vi "opc_client.vi"(8 "error in (no error)":errorcluster, 10 "server endpoint URL":string) -> (0 "error out":errorcluster, 1 "OPC UA client refnum out":T1, 2 "etat":string, 3 "temperature":dbl, 4 "Courant":dbl, 5 "Pression":dbl, 6 "Debit":dbl, 7 "Tension":dbl)   [LabVIEW 2019]
uses:
  <vilib>/OPCUA/controls/OPC UA Client Refnum.ctl
  <vilib>/OPCUA/controls/Time Out.ctl
  <vilib>/OPCUA/client/Multiple Read Variant.vi
  <vilib>/OPCUA/NI OPC UA Client.lvlib
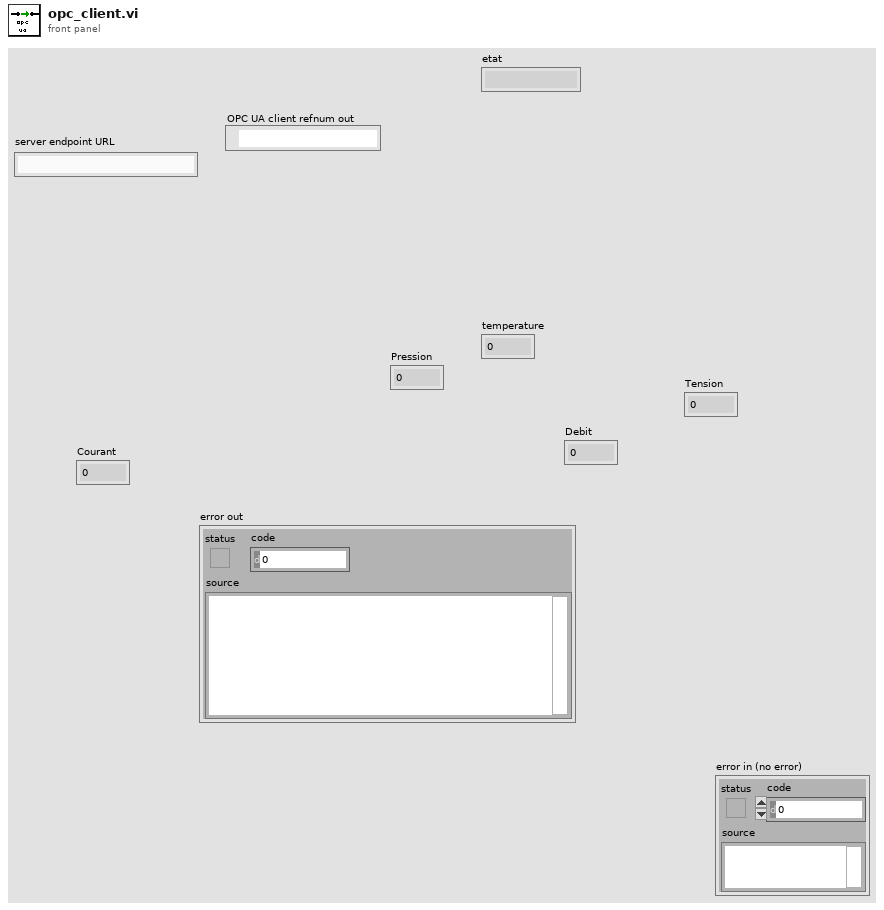
[diagram p1: front panel]
types:
  T1 = typedef "OPC UA Client Refnum.ctl" = refnum<k21>
  T2 = typedef "Time Out.ctl" = u32
  T3 = cluster{"message mode":enum16{"None", "Sign", "Sign and Encrypt"}, "security":enum16{"Basic256", "Basic128Rsa15"}}
  T4 = typedef "Read Variant Result.ctl" = cluster{"node ID":T5, "value ":variant, "timestamp":timestamp, "status":T6}
  T5 = typedef "NodeId.ctl" = string
  T6 = typedef "OPC UA StatusCode.ctl" = u32
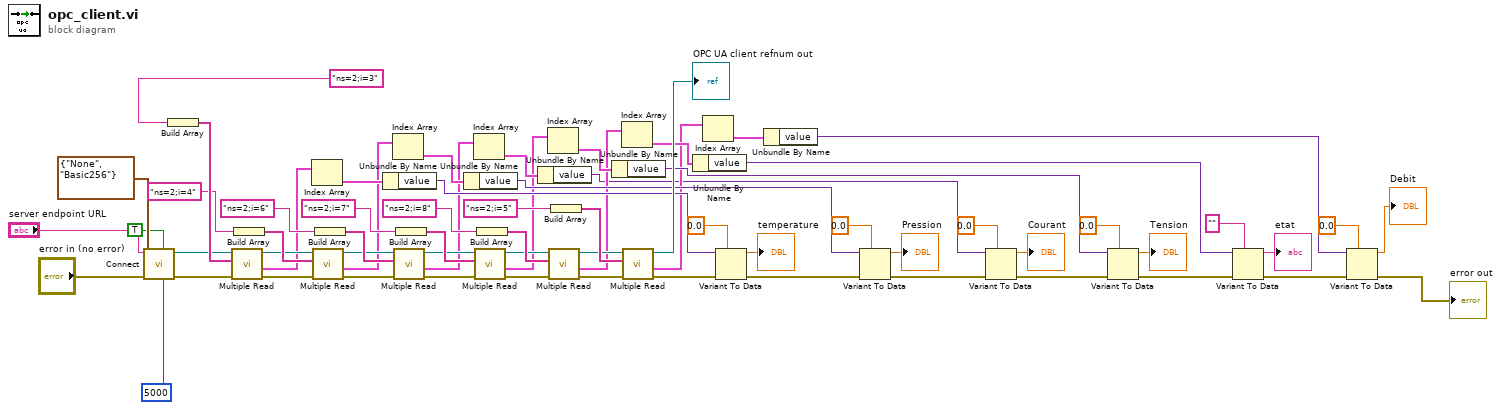
[diagram p0: block diagram]
diagram:
  n1 = call <vilib>:"Connect.vi"("timeout (5000 ms)"=T2 5000, "trust any server (F)"=TRUE, "error in (no error)"="error in (no error)", "security policy"=T3 {"message mode"=enum."None", "security"=enum."Basic256"}, "server endpoint URL"="server endpoint URL") -> ("error out"=w51:errorcluster, "OPC UA client refnum out"=w65:T1)  [unwired: 4 in, 1 out]
  n2 = Build Array("ns=2;i=3" ("ID")) -> (w66:string[])
  n3 = call-poly <vilib>:"Multiple Read.vi"("error in (no error)"=w51, "node IDs"=w66, "OPC UA client refnum in"=w65) -> ("error out"=w50:errorcluster, "results"=w40:T4[], "OPC UA client refnum out"=w57:T1)  [unwired: 5 in, 1 out]
  n4 = Build Array("ns=2;i=4" ("ID 6")) -> (w58:string[])
  n5 = Index Array(array=w40) -> (element=w39:T4)  [unwired: 1 in]
  n6 = call-poly <vilib>:"Multiple Read.vi"("error in (no error)"=w50, "node IDs"=w58, "OPC UA client refnum in"=w57) -> ("error out"=w49:errorcluster, "results"=w17:T4[], "OPC UA client refnum out"=w56:T1)  [unwired: 5 in, 1 out]
  n7 = Build Array("ns=2;i=6" ("ID 2")) -> (w62:string[])
  n8 = Unbundle By Name(w39) -> ("value"=w37:variant)
  n9 = Index Array(array=w17) -> (element=w21:T4)  [unwired: 1 in]
  n10 = call-poly <vilib>:"Multiple Read.vi"("error in (no error)"=w49, "node IDs"=w62, "OPC UA client refnum in"=w56) -> ("error out"=w48:errorcluster, "results"=w16:T4[], "OPC UA client refnum out"=w55:T1)  [unwired: 5 in, 1 out]
  n11 = Build Array("ns=2;i=7" ("ID 3")) -> (w61:string[])
  n12 = Unbundle By Name(w21) -> ("value"=w19:variant)
  n13 = Index Array(array=w16) -> (element=w32:T4)  [unwired: 1 in]
  n14 = call-poly <vilib>:"Multiple Read.vi"("error in (no error)"=w48, "node IDs"=w61, "OPC UA client refnum in"=w55) -> ("error out"=w47:errorcluster, "results"=w15:T4[], "OPC UA client refnum out"=w54:T1)  [unwired: 5 in, 1 out]
  n15 = Build Array("ns=2;i=8" ("ID 4")) -> (w60:string[])
  n16 = Unbundle By Name(w32) -> ("value"=w4:variant)
  n17 = Index Array(array=w15) -> (element=w29:T4)  [unwired: 1 in]
  n18 = call-poly <vilib>:"Multiple Read.vi"("error in (no error)"=w47, "node IDs"=w60, "OPC UA client refnum in"=w54) -> ("error out"=w46:errorcluster, "results"=w14:T4[], "OPC UA client refnum out"=w53:T1)  [unwired: 5 in, 1 out]
  n19 = Build Array("ns=2;i=5" ("ID 5")) -> (w59:string[])
  n20 = Unbundle By Name(w29) -> ("value"=w27:variant)
  n21 = Index Array(array=w14) -> (element=w35:T4)  [unwired: 1 in]
  n22 = call-poly <vilib>:"Multiple Read.vi"("error in (no error)"=w46, "node IDs"=w59, "OPC UA client refnum in"=w53) -> ("error out"=w6:errorcluster, "results"=w13:T4[], "OPC UA client refnum out"=→"OPC UA client refnum out":T1)  [unwired: 5 in, 1 out]
  n23 = Unbundle By Name(w35) -> ("value"=w34:variant)
  n24 = Index Array(array=w13) -> (element=w25:T4)  [unwired: 1 in]
  n25 = Variant To Data(error in=w6, type=0.0, Variant=w37) -> (data=→"temperature":dbl, error out=w5:errorcluster)
  n26 = Unbundle By Name(w25) -> ("value"=w23:variant)
  n27 = Variant To Data(error in=w5, type=0.0, Variant=w19) -> (data=→"Pression":dbl, error out=w11:errorcluster)
  n28 = Variant To Data(error in=w11, type=0.0, Variant=w4) -> (data=→"Courant":dbl, error out=w10:errorcluster)
  n29 = Variant To Data(error in=w10, type=0.0, Variant=w27) -> (data=→"Tension":dbl, error out=w9:errorcluster)
  n30 = Variant To Data(error in=w9, type="", Variant=w34) -> (data=→"etat":string, error out=w8:errorcluster)
  n31 = Variant To Data(error in=w8, type=0.0, Variant=w23) -> (data=→"Debit":dbl, error out=→"error out":errorcluster)
